vi "Destroy DSF Configuration Session.vi"(8 "error in (no error)":errorcluster, 11 "config data ref":T1) -> (0 "error out":errorcluster)   [LabVIEW 2017, in "DSF Core.lvlib" / "Configuration Session.lvclass"]
uses:
  Configuration Session.lvclass
  DSF Config Data Ref.ctl
  DSF Config Data.ctl
  Internal DSF Configuration.ctl
  Typedefs/DSF Version Info.ctl
  Internal DSF Plugin with ID.ctl
  Internal DSF Plugin Info.ctl
  Typedefs/DSF Timing Info.ctl
  Typedefs/DSF Engine Plugin Thread Configuration.ctl
  Typedefs/DSF Settings Info.ctl
  Internal DSF Group with ID.ctl
  Internal DSF Group Info.ctl
  Internal DSF Transfer with ID.ctl
  Internal DSF Transfer Info.ctl
  Internal DSF Channel with ID.ctl
  Internal DSF Channel Info.ctl
  Internal DSF Settings with ID.ctl
  Internal DSF Settings Info.ctl
  DSF Core.lvlib
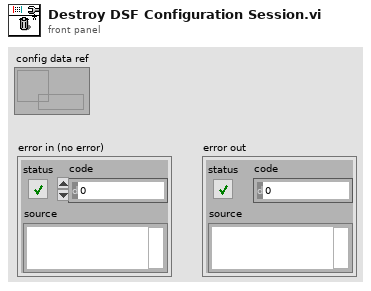
[diagram p1: front panel]
types:
  T1 = typedef "DSF Core.lvlib/Configuration Session.lvclass/DSF Config Data Ref.ctl" = refnum<data-value>
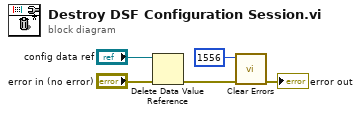
[diagram p0: block diagram]
diagram:
  n1 = Delete Data Value Reference(data value reference="config data ref", error in="error in (no error)") -> (error out=w5:errorcluster)  [unwired: 1 out]
  n2 = call <vilib>:"Clear Errors.vi"("error in (no error)"=w5, "specific error code to clear (0: all)"=1556) -> ("error out"=→"error out":errorcluster)  [unwired: 4 in, 1 out]
